vi "IsPointInsideField.vi"(8 "error in (no error)":errorcluster, 10 "Point":dbl[](array[numeric]), 11 "Field in":refnum<class "Field.lvclass">) -> (0 "error out":errorcluster, 2 "InsideField":bool=TRUE, 3 "Field out":refnum<class "Field.lvclass">)   [LabVIEW 2023, in "Field.lvclass"]
uses:
  Field.lvclass
  Field.lvclass/Field.ctl
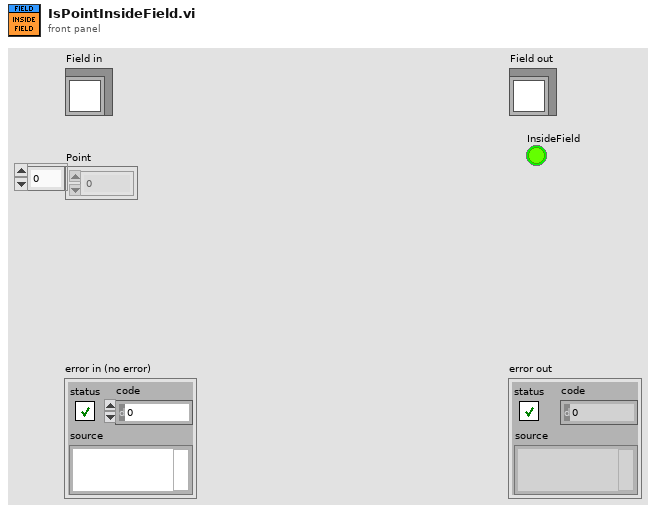
[diagram p1: front panel]
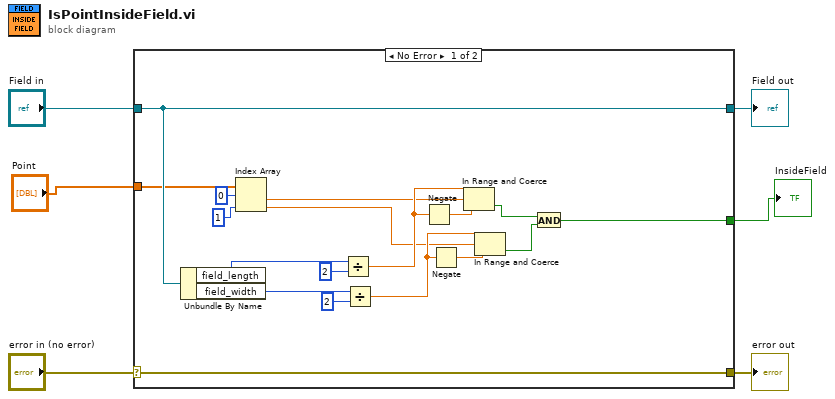
[diagram p0: block diagram]
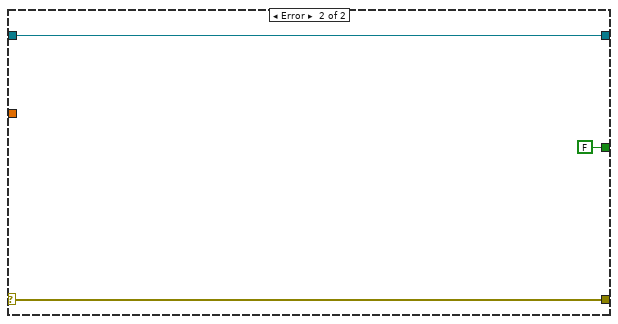
[diagram p2: hidden frame]
diagram:
  n1 = case shown="No Error" "error in (no error)" {
    selector: "error in (no error)" -> [w24 w27]
    tunnel: [w24 w27] -> w5
    tunnel: [w23 w26] -> w3
    tunnel: "Field in" -> [w23 w26]
    tunnel: "Point" -> [w18 _]
    tunnel: [w7 FALSE] -> w1
    frame No Error {
      n2 = Unbundle By Name(w23) -> ("field_length"=w22:i32, "field_width"=w11:i32)
      n3 = Index Array(array=w18, index #1=0 ("index"), index #2=1 ("index")) -> (element #1=w15:dbl, element #2=w10:dbl)
      n4 = Divide(x=w22, y=2) -> (x/y=w19:dbl)
      n5 = Divide(x=w11, y=2) -> (x/y=w14:dbl)
      n6 = Negate(x=w19) -> (-x=w20:dbl)
      n7 = Negate(x=w14) -> (-x=w13:dbl)
      n8 = In Range and Coerce(upper limit=w19, x=w15, lower limit=w20) -> (In Range?=w9:bool)  [unwired: 1 out]
      n9 = In Range and Coerce(upper limit=w14, x=w10, lower limit=w13) -> (In Range?=w8:bool)  [unwired: 1 out]
      n10 = And(x=w9, y=w8) -> (x .and. y?=w7:bool)
    }
    frame Error {
    }
  }
  "error out" <- w5
  "Field out" <- w3
  "InsideField" <- w1
